vi "CRC.vi"() -> (3 "CRC16":u16 format="%x")   [LabVIEW 2009]
uses:
  CRCDLL.dll
panel:
  in  "字符串":string
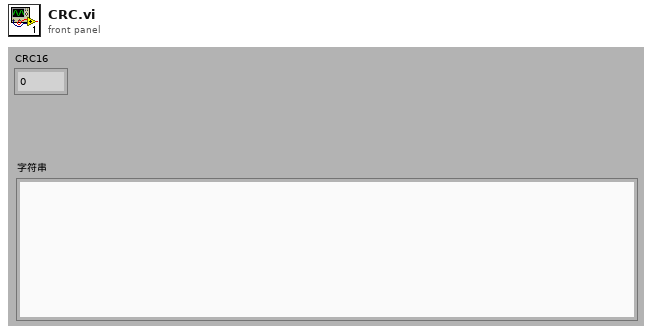
[diagram p1: front panel]
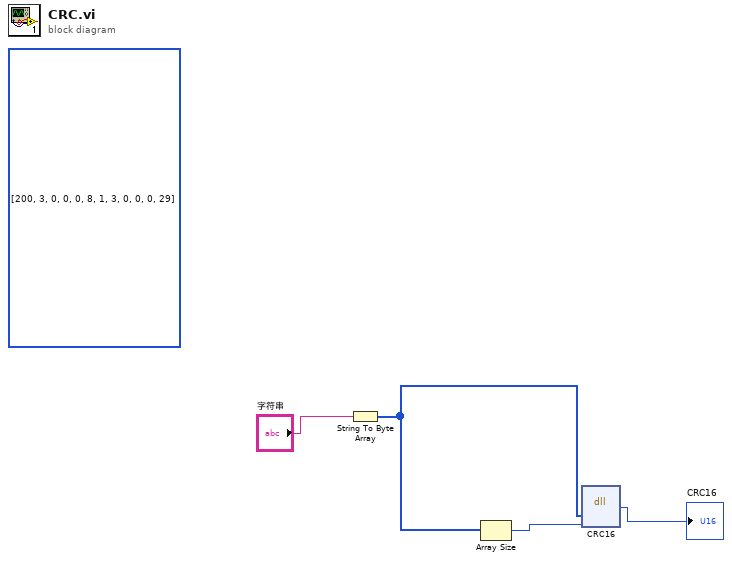
[diagram p0: block diagram]
diagram:
  (unwired) u8[] [200, 3, 0, 0, 0, 8, 1, 3, 0, 0, 0, 29] ("puchMsg")
  n1 = String To Byte Array(string="字符串") -> (unsigned byte array=w1:u8[])
  n2 = Array Size(array=w1) -> (size(s)=w4:i32)
  n3 = dll-call lib="E:/luyuanshan/Powerwise/上位机/GPRS监控/远程监控中心/SubVi/CRCDLL.dll" fn="CRC16"("参数1"=w1, "参数2"=w4) -> ("返回类型"=→"CRC16":i32)  [unwired: 4 in, 3 out]
